vi "CMI About Dialog.vi"(9 "E-mail:":string="author@email.com", 10 "Author:":string="author", 11 "Title":string="application title") -> ()   [LabVIEW 2020, in "varilib.lvlib"]
doc: "Shows application about dialog for Czech Metrology Institute"
uses:
  varilib.lvlib
panel:
  out "copyright":string="author"
  in  "OK":bool
  out "address":string="Czech Metrology Institute\nDepartment 6011, DC and LF electrical quantities\nOkružní 31\n63800, Brno\nCzech Republic"
  out "www:":string="http://www.cmi.cz"
  out "Version:":string
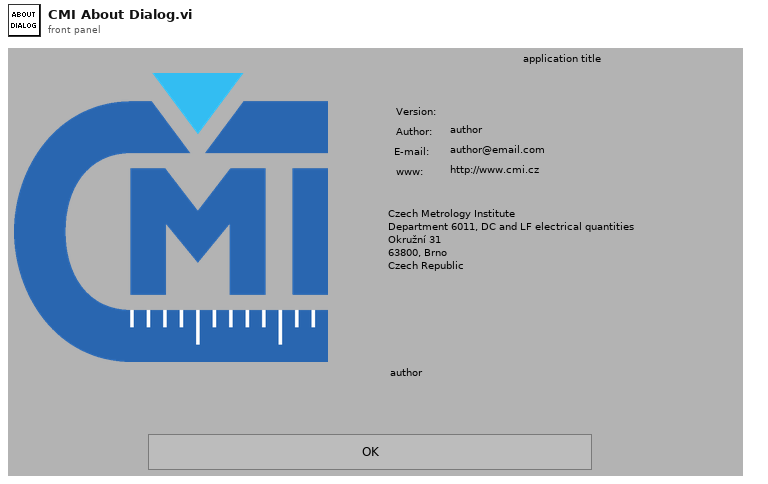
[diagram p1: front panel]
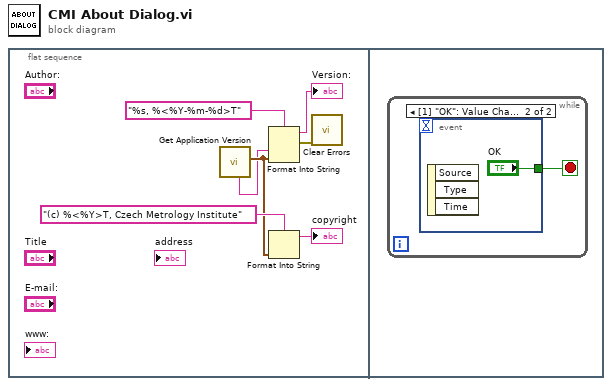
[diagram p0: block diagram]
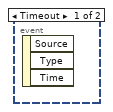
[diagram p2: hidden frame]
diagram:
  n1 = flat-sequence {
    frame #0 {
      n2 = call "Get Application Version.vi"() -> ("exe file last modification"=w2:timestamp, "version number string"=w1:string)  [unwired: 8 in, 2 out]
      n3 = Format Into String(format string="%s, %<%Y-%m-%d>T" ("time format string (%c)"), w1, w2) -> (resulting string=→"Version:":string, error out=w6:errorcluster)  [unwired: 2 in]
      n4 = Format Into String(format string="(c) %<%Y>T, Czech Metrology Institute", w2) -> (resulting string=→"copyright":string)  [unwired: 2 in, 1 out]
      n5 = call <vilib>:"Clear Errors.vi"("error in (no error)"=w6) -> ()  [unwired: 5 in, 2 out]
    }
    frame #1 {
      n6 = while {
        stop <- w8 stop-if-true
        n7 = event shown="[1] \"OK\": Value Change;  Panel Close" {
          selector: _ -> [_ _]
          dyn-events: _ -> [_ _]
          timeout: _ -> [_ _]
          tunnel: [_ "OK"] -> w8
          event Timeout {
            n8 = event-data() -> ()  [unwired: 1 in, 3 out]
          }
          event "OK": Value Change; Panel Close {
            n9 = event-data() -> ()  [unwired: 1 in, 3 out]
          }
        }
      }
    }
  }
